vi "Task.vi"() -> ()   [LabVIEW 2024]
uses:
  <vilib>/DAQmx/read.llb/DAQmx Read (Analog 1D Wfm NChan NSamp).vi
  <vilib>/DAQmx/miscellaneous.llb/DAQmx Fill In Error Info.vi
  <vilib>/Utility/file.llb/Write Delimited Spreadsheet (DBL).vi
panel:
  out "new file path (Not A Path if cancelled) 2":path
  out "data":waveform(dbl)[](graph)
  in  "stop":bool
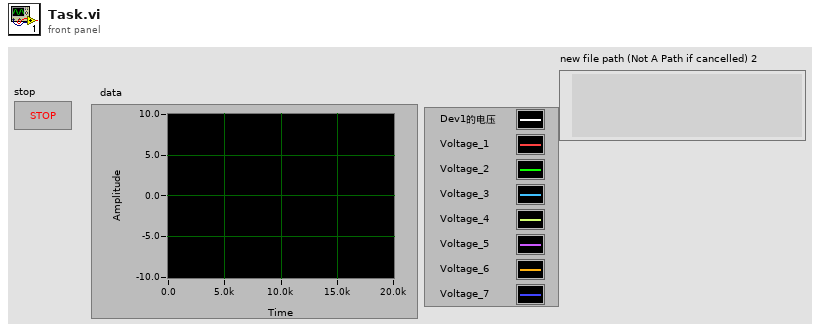
[diagram p1: front panel]
types:
  T1 = enum16{"open", "open or create", "create or replace", "create", "open (read-only)"}
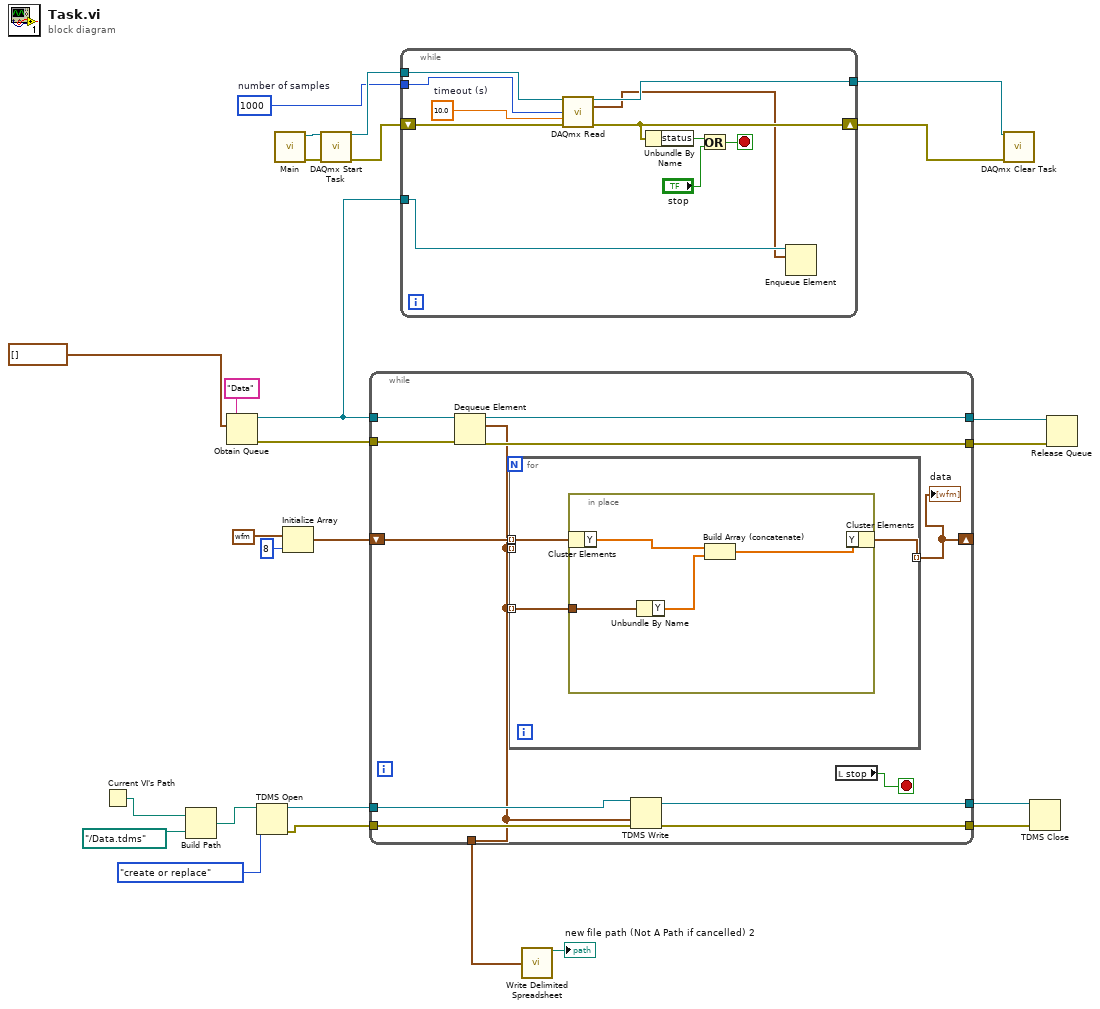
[diagram p0: block diagram]
diagram:
  w24 = 1000  # number of samples
  n1 = Current VI's Path() -> (path=w9:path)
  n2 = Build Path(base path=w9, name or relative path=path "../Data.tdms") -> (appended path=w7:path)
  n3 = Obtain Queue(name (unnamed)="Data", element data type=waveform(dbl)[] [] ("data")) -> (queue out=w16:refnum<queue>, error out=w17:errorcluster)  [unwired: 3 in, 1 out]
  n4 = TDMS Open(10:T1."create or replace" ("operation (0:open)"), 11:w7) -> (0:w5:errorcluster, 3:w10:refnum<k34>)  [unwired: 5 in]
  n5 = call "Main.vi"() -> ("error out"=w20:errorcluster, "task out"=w21:refnum<k21>)  [unwired: 10 in]
  n6 = Initialize Array(waveform(dbl) {"t0"=timestamp(0 s since 1904-01-01), "dt"=0.0, "Y"=[]} ("data"), 8 ("dimension size")) -> (w11:waveform(dbl)[])
  n7 = call <vilib>:"DAQmx Start Task.vi"("task/channels in"=w21, "error in"=w20) -> ("task out"=w26:refnum<k21>, "error out"=w25:errorcluster)  [unwired: 12 in]
  n8 = while {
    tunnel: w17 -> [w38]
    tunnel: w16 -> [w37]
    tunnel: [w36] -> w15
    tunnel: [w35] -> w14
    shift-right: [w32] -> _
    shift-left: w11 -> [w33]
    tunnel: w10 -> [w31]
    tunnel: w5 -> [w30]
    tunnel: [w29] -> w4
    tunnel: [w28] -> w3
    tunnel: [w27] -> w2
    stop <- w34 stop-if-true
    n9 = Dequeue Element(queue=w37, error in (no error)=w38) -> (queue out=w36:refnum<queue>, element=w27:waveform(dbl)[], error out=w35:errorcluster)  [unwired: 1 in, 1 out]
    n10 = for {
      tunnel: w27 -> [_] mode=indexing
      tunnel: w33 -> [w41] mode=indexing
      tunnel: [w40] -> w32 mode=indexing
      tunnel: w27 -> [w39] mode=indexing
      n11 = in-place {
        in-place-border: w39 -> [w43]
        n12 = in-place-cluster #1(w41) -> ("Y"=w45:dbl[])
        n13 = Unbundle By Name(w43) -> ("Y"=w42:dbl[])
        n14 = Build Array (concatenate)(w45, w42) -> (w44:dbl[])
        n15 = in-place-cluster #1("Y"=w44) -> (w40:waveform(dbl))
      }
    }
    "data" <- w32
    n16 = TDMS Write(0:w31, 9:w27, 11:w30) -> (4:w29:refnum<k34>, 15:w28:errorcluster)  [unwired: 3 in, 2 out]
    n17 = local read "stop"() -> (w34:bool)
  }
  n18 = while {
    tunnel: w26 -> [w56]
    tunnel: w24 -> [w53]
    tunnel: [w54] -> w22
    shift-right: [w51] -> w23
    shift-left: w25 -> [w55]
    tunnel: w16 -> [w47]
    stop <- w50 stop-if-true
    w48 = 10.0  # timeout (s)
    n19 = call-poly <vilib>:"DAQmx Read.vi"("task/channels in"=w56, "number of samples per channel"=w53, "timeout"=w48, "error in"=w55) -> ("task out"=w54:refnum<k21>, "data"=w46:waveform(dbl)[], "error out"=w51:errorcluster)  [unwired: 9 in]
    n20 = Unbundle By Name(w51) -> ("status"=w52:bool)
    n21 = Or(x=w52, y="stop") -> (x .or. y?=w50:bool)
    n22 = Enqueue Element(queue=w47, element=w46) -> ()  [unwired: 2 in, 3 out]
  }
  n23 = call-poly <vilib>:"Write Delimited Spreadsheet.vi"("1D data"=w2) -> ("new file path (Not A Path if cancelled)"=→"new file path (Not A Path if cancelled) 2":path)  [unwired: 13 in, 1 out]
  n24 = call <vilib>:"DAQmx Clear Task.vi"("task in"=w22, "error in"=w23) -> ()  [unwired: 13 in, 1 out]
  n25 = TDMS Close(8:w3, 11:w4) -> ()  [unwired: 2 out]
  n26 = Release Queue(queue=w15, error in (no error)=w14) -> ()  [unwired: 1 in, 3 out]
